vi "tearDown.vi"(8 "error in (no error)":errorcluster, 11 "reference in":refnum<class "Scan Engine Scripting API Custom Device Unit Tests.lvclass">) -> (0 "error out":errorcluster, 3 "reference out":refnum<class "Scan Engine Scripting API Custom Device Unit Tests.lvclass">)   [LabVIEW 2019, in "Scan Engine Scripting API Custom Device Unit Tests.lvclass"]
doc: "tearDown runs after the test method has completed. Use this method to clean up any operations or references that were opened by setUp or the test method. Unit tests should be independent of other unit tests so this VI should ensure that the next test can run in a 'clean' test environment."
uses:
  Scan Engine Scripting API Custom Device Unit Tests.lvclass
  Scan Engine Scripting API Custom Device Unit Tests.lvclass/Scan Engine Scripting API Custom Device Unit Tests.ctl
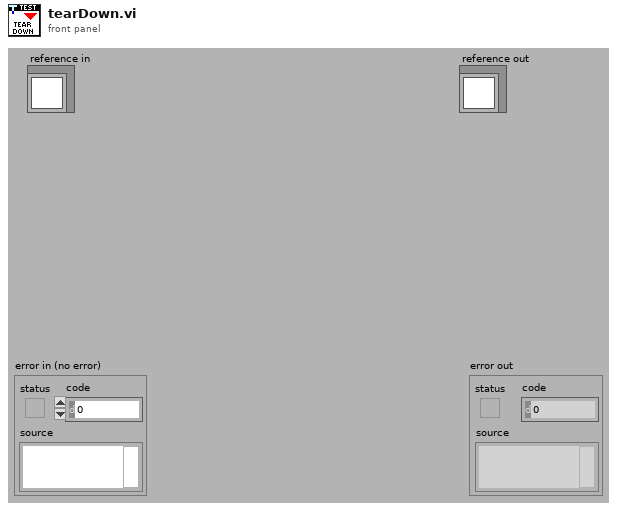
[diagram p1: front panel]
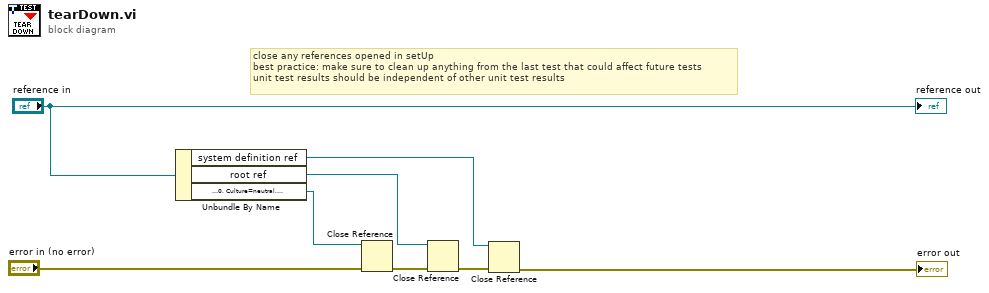
[diagram p0: block diagram]
diagram:
  # "close any references opened in setUp\nbest practice: make sure to clean up anything from the last test that could affect future tests\nunit test results should be independent of other unit test results"
  n1 = Unbundle By Name("reference in") -> ("system definition ref"=w4:refnum<k24>, "root ref"=w5:refnum<k24>, "target ref"=w6:refnum<k24>)
  n2 = Close Reference(reference=w6, error in (no error)="error in (no error)") -> (error out=w7:errorcluster)
  n3 = Close Reference(reference=w5, error in (no error)=w7) -> (error out=w3:errorcluster)
  n4 = Close Reference(reference=w4, error in (no error)=w3) -> (error out=→"error out":errorcluster)
  "reference out" <- "reference in"
